vi "HT3_Write.vi"(7 "Apend":bool, 8 "error in":errorcluster, 9 "Data Count":i32, 10 "Data in":u32[](array[numeric]), 11 "refnum in":refnum<file>) -> (0 "error out":errorcluster, 3 "refnum out":refnum<file>)   [LabVIEW 2009]
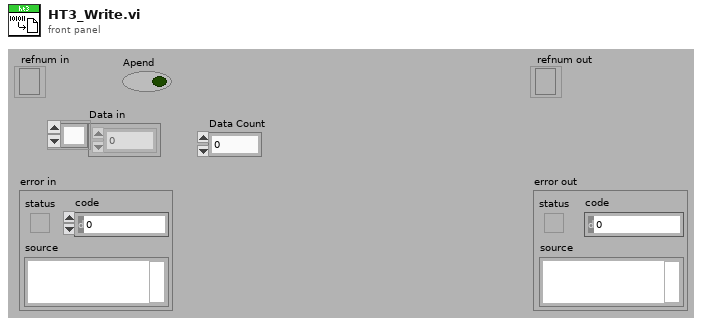
[diagram p1: front panel]
types:
  T1 = enum16{"big-endian, network order", "native, host order", "little-endian"}
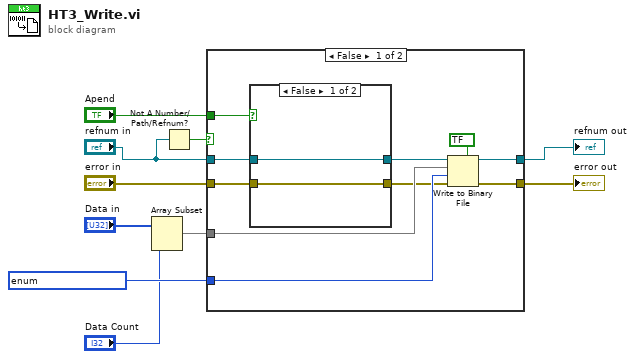
[diagram p0: block diagram]
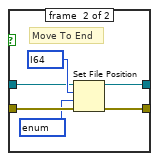
[diagram p2: hidden frame]
diagram:
  n1 = Array Subset(array="Data in", length="Data Count") -> (w2:u32[])  [unwired: 1 in]
  n2 = Not A Number/Path/Refnum?(number/path/refnum="refnum in") -> (NaN/Path/Refnum?=w4:bool)
  n3 = case shown="False" w4 {
    tunnel: "error in" -> [w20 w30]
    tunnel: "refnum in" -> [w19 w29]
    tunnel: T1 ? ("byte order (0:big-endian, network order)") -> [w18 _]
    tunnel: "Apend" -> [w17 _]
    tunnel: [w16 w29] -> w7
    tunnel: w2 -> [w15 _]
    tunnel: [w14 w30] -> w6
    frame #0 {
      n4 = case shown="False" w17 {
        tunnel: w20 -> [w22 w27]
        tunnel: w19 -> [w21 w26]
        tunnel: [w22 w24] -> w13
        tunnel: [w21 w23] -> w12
        frame #0 {
        }
        frame #1 {
          # "Move To End"
          n5 = Set File Position(offset (in bytes) (0)=i64 ?, refnum=w26, from (0:start)=enum16{"start", "end", "current"} ?, error in=w27) -> (refnum out=w23:refnum<file>, error out=w24:errorcluster)
        }
      }
      n6 = Write to Binary File(file (use dialog)=w12, data=w15, error in=w13, 5:bool ? ("prepend array or string size? (T)"), 9:w18) -> (refnum out=w16:refnum<file>, error out=w14:errorcluster)  [unwired: 2 out]
    }
    frame #1 {
    }
  }
  "refnum out" <- w7
  "error out" <- w6
